vi "Multi Write.vi"(7 "Datas":i32[](array[numeric]), 8 "error in (no error)":errorcluster, 10 "Start Register":i32, 11 "Slave Address":i32) -> (0 "error out":errorcluster, 2 "Command":string)   [LabVIEW 2014, in "Modbus.lvlib"]
uses:
  Modbus.lvlib
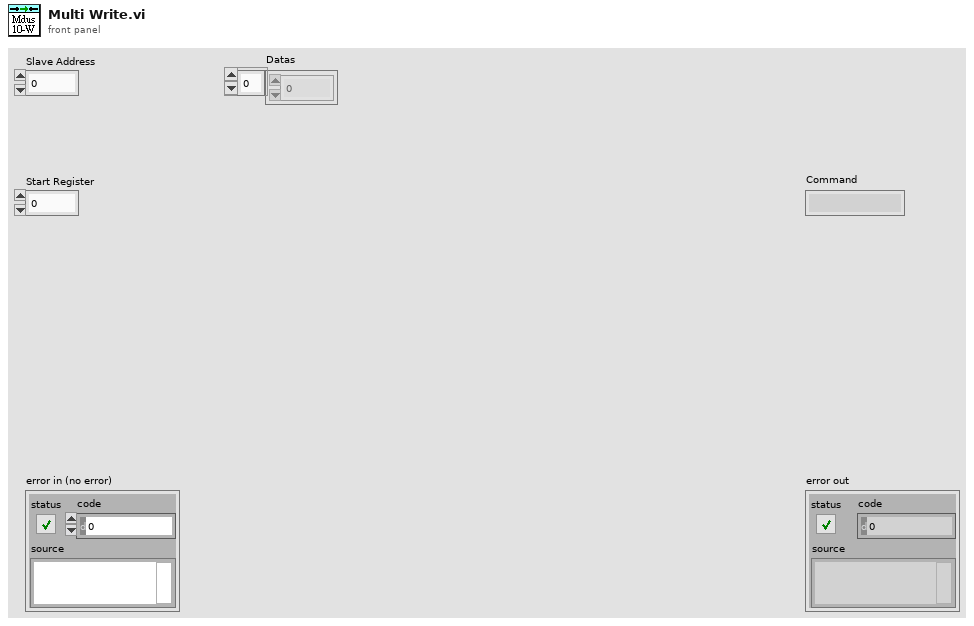
[diagram p1: front panel]
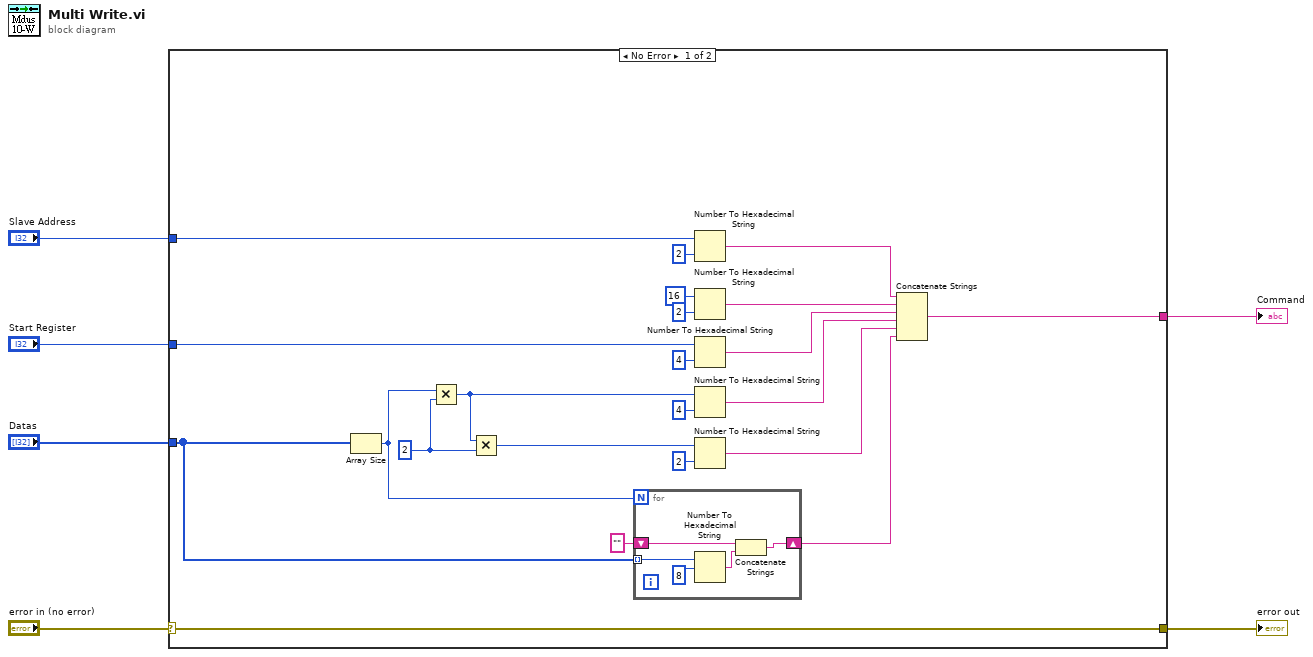
[diagram p0: block diagram]
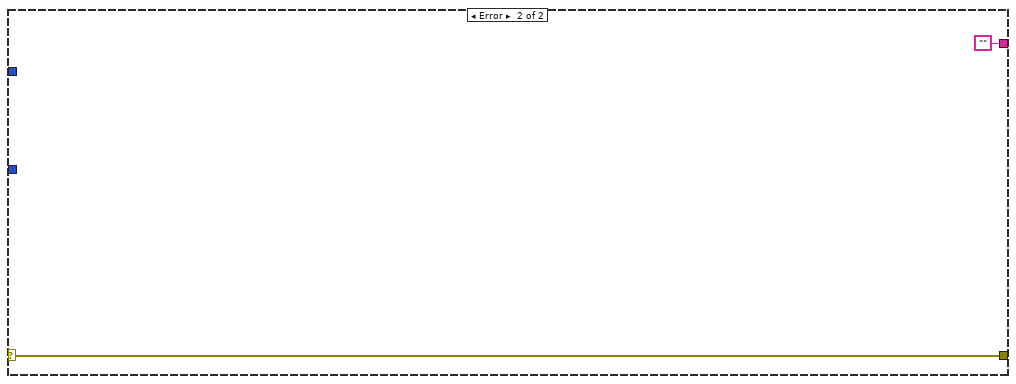
[diagram p2: hidden frame]
diagram:
  n1 = case shown="No Error" "error in (no error)" {
    selector: "error in (no error)" -> [w28 w35]
    tunnel: [w28 w35] -> w5
    tunnel: "Slave Address" -> [w9 _]
    tunnel: "Start Register" -> [w8 _]
    tunnel: [w10 ""] -> w2
    tunnel: "Datas" -> [w7 _]
    frame No Error {
      w15 = 2 ("y")
      n2 = Array Size(array=w7) -> (size(s)=w12:i32)
      n3 = Multiply(x=w12, y=w15) -> (x*y=w13:i32)
      n4 = Multiply(x=w13, y=w15) -> (x*y=w14:i32)
      n5 = for {
        N: w12 -> [_]
        tunnel: w7 -> [w32] mode=indexing
        shift-right: [w31] -> w18
        shift-left: "" -> [w30]
        n6 = Number To Hexadecimal String(1:i16 8 ("width (-)"), 2:w32) -> (0:w29:string)
        n7 = Concatenate Strings(w30, w29) -> (w31:string)
      }
      n8 = Number To Hexadecimal String(1:i16 2 ("width (-)"), 2:w9) -> (0:w11:string)
      n9 = Number To Hexadecimal String(1:i16 2 ("width (-)"), 2:16 ("number")) -> (0:w22:string)
      n10 = Number To Hexadecimal String(1:i16 4 ("width (-)"), 2:w8) -> (0:w21:string)
      n11 = Number To Hexadecimal String(1:i16 4 ("width (-)"), 2:w13) -> (0:w16:string)
      n12 = Number To Hexadecimal String(1:i16 2 ("width (-)"), 2:w14) -> (0:w17:string)
      n13 = Concatenate Strings(w11, w22, w21, w16, w17, w18) -> (w10:string)
    }
    frame Error {
    }
  }
  "error out" <- w5
  "Command" <- w2
